vi "check-status.vi"(10 "warning":bool, 11 "error":bool) -> (0 "msg":string, 1 "status":u32, 2 "warning_out":bool, 3 "error_out":bool)   [LabVIEW 2014]
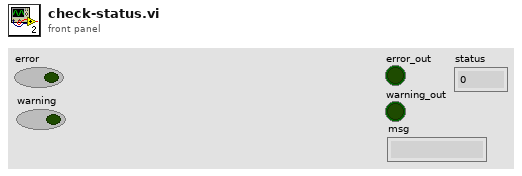
[diagram p1: front panel]
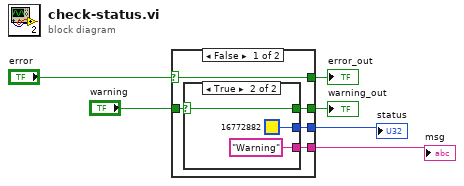
[diagram p0: block diagram]
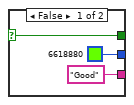
[diagram p2: hidden frame]
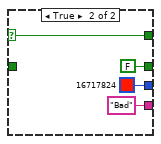
[diagram p3: hidden frame]
diagram:
  n1 = case shown="False" "error" {
    selector: "error" -> [w9 w20]
    tunnel: "warning" -> [w11 _]
    tunnel: [w10 u32 16717824] -> w2
    tunnel: [w9 w20] -> w4
    tunnel: [w8 FALSE] -> w3
    tunnel: [w7 "Bad"] -> w1
    frame False {
      n2 = case shown="True" w11 {
        selector: w11 -> [w13 w16]
        tunnel: [u32 6618880 u32 16772882] -> w10
        tunnel: [w13 w16] -> w8
        tunnel: ["Good" "Warning"] -> w7
        frame False {
        }
        frame True {
        }
      }
    }
    frame True {
    }
  }
  "error_out" <- w4
  "warning_out" <- w3
  "status" <- w2
  "msg" <- w1
